vi "Set to Discovery Mode.vi"(11 "IED in":refnum<class "IED.lvclass">) -> (3 "IED out":refnum<class "IED.lvclass">)   [LabVIEW 2018, in "IED Actor.lvlib" / "IED.lvclass"]
uses:
  IED.lvclass
  IED.lvclass/IED.ctl
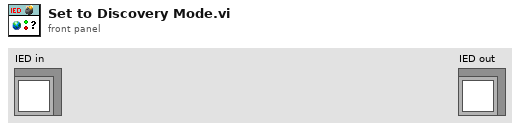
[diagram p1: front panel]
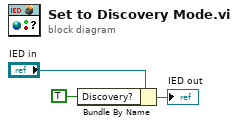
[diagram p0: block diagram]
diagram:
  n1 = Bundle By Name(cluster="IED in", "Discovery?"=TRUE) -> (→"IED out":refnum<class "IED.lvclass">)
